vi "toml_value_float.vi"(5 "operation":T1, 7 "section":string[](array[string]), 8 "error in (no error)":errorcluster, 9 "value in":dbl, 10 "key":string[](array[string]), 11 "path in":path) -> (0 "error out":errorcluster, 1 "value out":dbl, 2 "exists?":bool, 3 "path out":path)   [LabVIEW 2017]
uses:
  toml_value_operation.ctl
  toml_fg_action.ctl
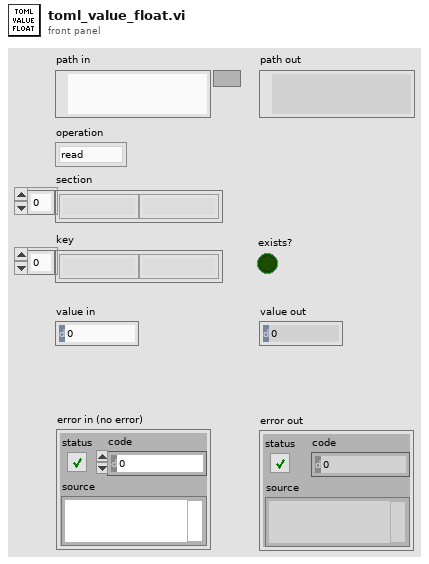
[diagram p1: front panel]
types:
  T1 = typedef "toml_value_operation.ctl" = enum8{"read", "write", "delete"}
  T2 = typedef "toml_fg_action.ctl" = enum8{"null", "get", "set", "pop", "import", "export", "drop"}
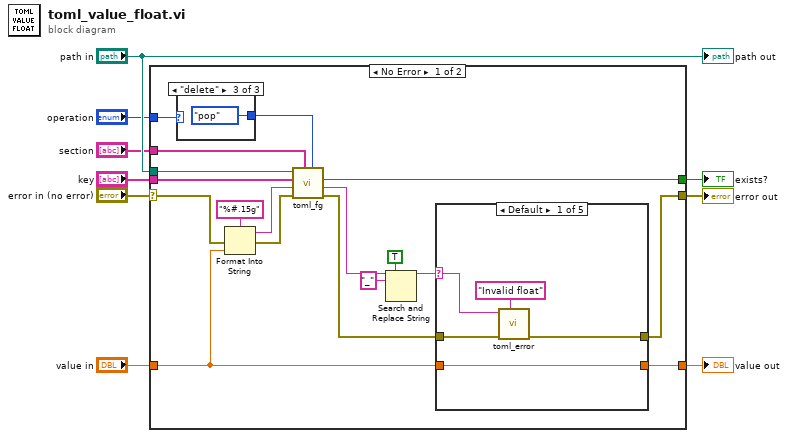
[diagram p0: block diagram]
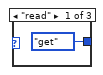
[diagram p2: hidden frame]
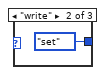
[diagram p3: hidden frame]
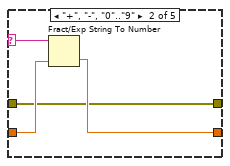
[diagram p4: hidden frame]
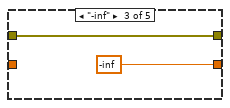
[diagram p5: hidden frame]
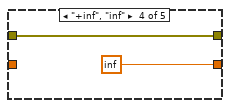
[diagram p6: hidden frame]
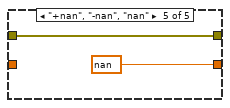
[diagram p7: hidden frame]
diagram:
  n1 = case shown="No Error" "error in (no error)" {
    selector: "error in (no error)" -> [w11 w47]
    tunnel: [w19 w47] -> w8
    tunnel: "path in" -> [w27 _]
    tunnel: "operation" -> [w25 _]
    tunnel: "section" -> [w24 _]
    tunnel: "key" -> [w23 _]
    tunnel: [w22 _] -> w3
    tunnel: [w21 w46] -> w2
    tunnel: "value in" -> [w18 w46]
    frame No Error {
      n2 = case shown="\"delete\"" w25 {
        tunnel: [toml_fg_action."get" ("action") toml_fg_action."set" ("action") toml_fg_action."pop" ("action")] -> w26
        frame "read" {
        }
        frame "write" {
        }
        frame "delete" {
        }
      }
      n3 = Format Into String(format string="%#.15g", error in=w11, w18) -> (resulting string=w17:string, error out=w10:errorcluster)  [unwired: 1 in]
      n4 = call "toml_fg.vi"("action"=w26, "section"=w24, "error in (no error)"=w10, "value in"=w17, "key"=w23, "path in"=w27) -> ("error out"=w20:errorcluster, "value out"=w16:string, "exists?"=w22:bool)  [unwired: 2 in, 1 out]
      n5 = Search and Replace String(replace all?=TRUE ("replace all? (F)"), input string=w16, search string="_") -> (result string=w15:string)  [unwired: 5 in, 3 out]
      n6 = case shown="Default" w15 {
        selector: w15 -> [w31 w39 _ _ _]
        tunnel: [w32 w37 -inf ("value in") inf ("value in") nan ("value in")] -> w21
        tunnel: [w34 w36 w40 w42 w44] -> w19
        tunnel: w20 -> [w35 w36 w40 w42 w44]
        tunnel: w18 -> [w32 w38 _ _ _]
        frame Default {
          n7 = call "toml_error.vi"("message"="Invalid float", "error in (no error)"=w35, "toml"=w31) -> ("error out"=w34:errorcluster)  [unwired: 8 in]
        }
        frame "+", "-", "0".."9" {
          n8 = Fract/Exp String To Number(string=w39, default (0 dbl)=w38) -> (number=w37:dbl)  [unwired: 2 in, 1 out]
        }
        frame "-inf" {
        }
        frame "+inf", "inf" {
        }
        frame "+nan", "-nan", "nan" {
        }
      }
    }
    frame Error {
    }
  }
  "error out" <- w8
  "value out" <- w2
  "exists?" <- w3
  "path out" <- "path in"
